vi "1D Array zusammenstutzen.vi"(6 "Speicher Freigeben":bool, 8 "error in (no error)":errorcluster caption="Fehler (Eingang, kein Fehler)", 10 "Anzahl Elemente":i32, 11 "Messdaten":sgl[](array[numeric])) -> (0 "error out":errorcluster caption="Fehler (Ausgang)", 3 "Messdaten":sgl[](array[numeric]))   [LabVIEW 2020, in "Linearisierung v2.lvlib"]
uses:
  Linearisierung v2.lvlib
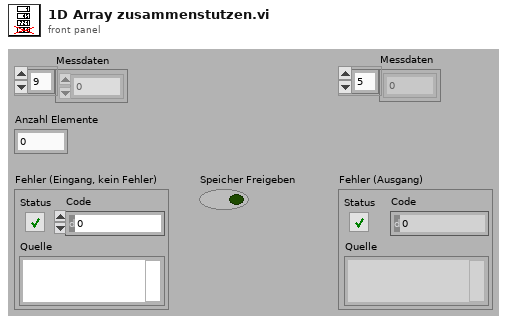
[diagram p1: front panel]
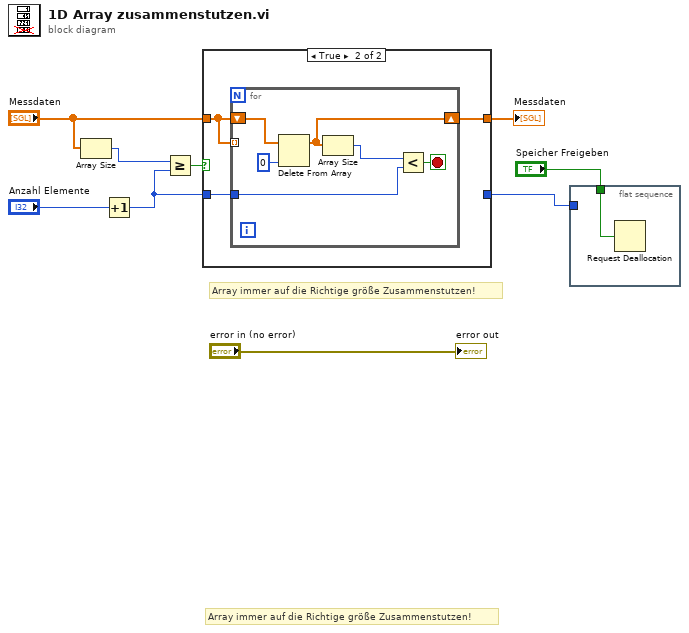
[diagram p0: block diagram]
diagram:
  # "Array immer auf die Richtige größe Zusammenstutzen!"
  # "Array immer auf die Richtige größe Zusammenstutzen!"
  n1 = Array Size(array="Messdaten") -> (size(s)=w3:i32)
  n2 = Increment(x="Anzahl Elemente") -> (x+1=w2:i32)
  n3 = Greater Or Equal?(x=w3, y=w2) -> (x >= y?=w9:bool)
  n4 = case shown="True" w9 {
    tunnel: "Messdaten" -> [w11 w13]
    tunnel: [w11 w12] -> w7
    tunnel: w2 -> [w10 w14]
    tunnel: [w10 _] -> w5
    frame False {
    }
    frame True {
      n5 = for {
        tunnel: w14 -> [w19]
        tunnel: w13 -> [_] mode=indexing
        shift-right: [w16] -> w12
        shift-left: w13 -> [w20]
        stop <- w18 stop-if-true
        n6 = Delete From Array(array=w20, index=0 ("Index")) -> (array with subset deleted=w16:sgl[])  [unwired: 1 in, 1 out]
        n7 = Array Size(array=w16) -> (size(s)=w15:i32)
        n8 = Less?(x=w15, y=w19) -> (x < y?=w18:bool)
      }
    }
  }
  "Messdaten" <- w7
  n9 = flat-sequence {
    tunnel: w5 -> [_]
    tunnel: "Speicher Freigeben" -> [w21]
    frame #0 {
      n10 = Request Deallocation(w21) -> ()
    }
  }
  "error out" <- "error in (no error)"
